vi "HSCAN.vi"(0 "refnum in":refnum<vi>, 1 "Cursor":string, 2 "Key":string, 5 "Use Pattern ?":bool, 7 "Pattern":string, 11 "error in":errorcluster, 12 "Use Count ?":bool, 13 "Count":string) -> (4 "refnum out":refnum<vi>, 6 "Data":T1, 15 "error out":errorcluster)   [LabVIEW 2023]
uses:
  SubVIs/Controls/redis-data.ctl
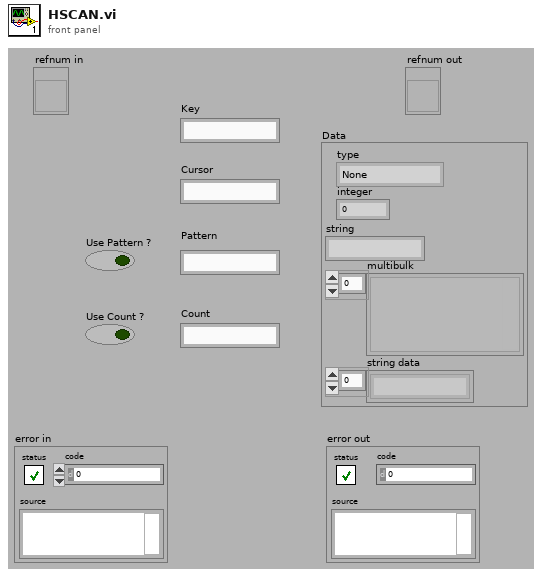
[diagram p1: front panel]
types:
  T1 = typedef "redis-data.ctl" = cluster{"type":enum16{"None", "Error", "Status", "Nil", "Integer", "String", "Multibulk"}, "integer":i64, "string":string, "multibulk":variant[], "string data":string[]}
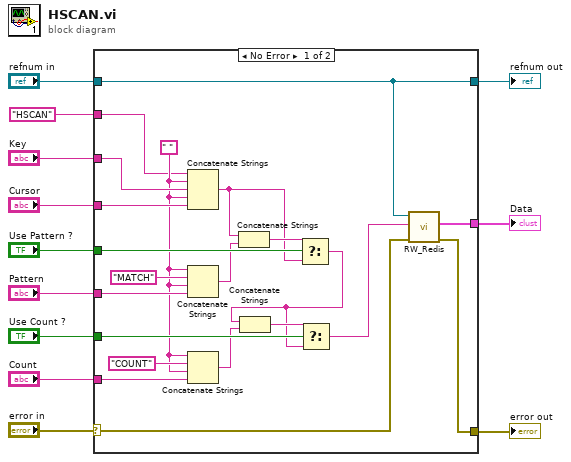
[diagram p0: block diagram]
diagram:
  n1 = case shown="No Error" "error in" {
    selector: "error in" -> [w33 w35]
    tunnel: "Cursor" -> [w30 _]
    tunnel: "HSCAN" -> [w13 _]
    tunnel: "refnum in" -> [w16 w34]
    tunnel: [w32 w35] -> w10
    tunnel: [w31 _] -> w2
    tunnel: "Pattern" -> [w29 _]
    tunnel: "Use Pattern ?" -> [w27 _]
    tunnel: "Use Count ?" -> [w20 _]
    tunnel: "Count" -> [w25 _]
    tunnel: [w16 w34] -> w4
    tunnel: "Key" -> [w15 _]
    frame No Error {
      w14 = " "
      n2 = Concatenate Strings(w13, w14, w15, w14, w30) -> (w23:string)
      n3 = Concatenate Strings(w14, "MATCH", w14, w29) -> (w22:string)
      n4 = Concatenate Strings(w14, "COUNT", w14, w25) -> (w18:string)
      n5 = Concatenate Strings(w23, w22) -> (w24:string)
      n6 = Select(t=w24, s=w27, f=w23) -> (s? t:f=w19:string)
      n7 = Concatenate Strings(w19, w18) -> (w21:string)
      n8 = Select(t=w21, s=w20, f=w19) -> (s? t:f=w17:string)
      n9 = call "RW_Redis.vi"("error in"=w33, "command"=w17, "refnum"=w16) -> ("error out"=w32:errorcluster, "Data"=w31:T1)  [unwired: 7 in]
    }
    frame Error {
    }
  }
  "error out" <- w10
  "Data" <- w2
  "refnum out" <- w4
